vi "RSZVB Response Cleanup.vi"(1 "Input String":string) -> (0 "Output String":string)   [LabVIEW 2010]
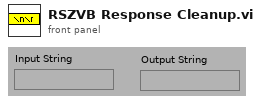
[diagram p1: front panel]
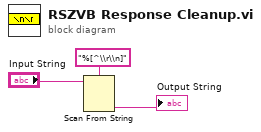
[diagram p0: block diagram]
diagram:
  n1 = Scan From String(format string="%[^\\r\\n]", input string="Input String") -> (output 1=→"Output String":string)  [unwired: 3 in, 3 out]
